vi "fgv_pf-val.vi"(7 "cmd":T4, 11 "pf-val":T3={"DT"=0.0, "SIM_TIME"=0.0, "MAX_RANGE"=0.0, "NP"=0, "NTh"=0, "Q_sim"=[[0.04000000000000001]], "R_sim"=[[1.0, 0.0], [0.0, 0.2741556778080377]]}) -> (3 "pf-val out":T2={"DT"=0.0, "SIM_TIME"=0.0, "MAX_RANGE"=0.0, "NP"=0, "NTh"=0.0, "Q_sim"=[[0.04000000000000001]], "R_sim"=[[1.0, 0.0], [0.0, 0.2741556778080377]]})   [LabVIEW 2019]
uses:
  Ctrl/cmd_common.ctl
  <vilib>/Analysis/Matrix/Datatypes/RealMatrix.ctl
  <vilib>/Analysis/Matrix/NI_Matrix.lvlib
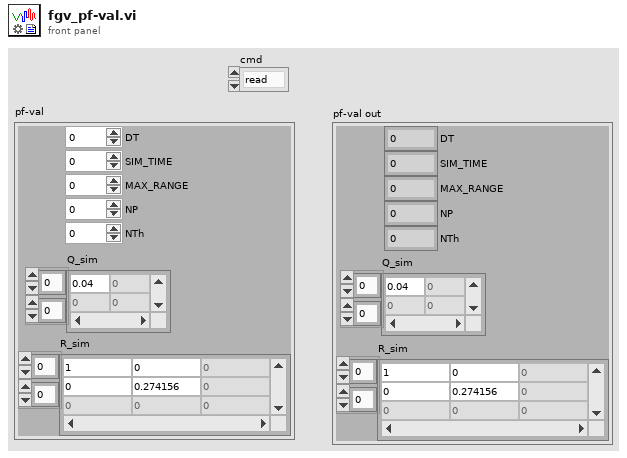
[diagram p1: front panel]
types:
  T1 = typedef "NI_Matrix.lvlib/RealMatrix.ctl" = dbl[][]
  T2 = cluster{"DT":dbl, "SIM_TIME":dbl, "MAX_RANGE":dbl, "NP":u32, "NTh":dbl, "Q_sim":T1, "R_sim":T1}
  T3 = cluster{"DT":dbl, "SIM_TIME":dbl, "MAX_RANGE":dbl, "NP":u32, "NTh":u32, "Q_sim":T1, "R_sim":T1}
  T4 = typedef "cmd_common.ctl" = enum16{"read", "write"}
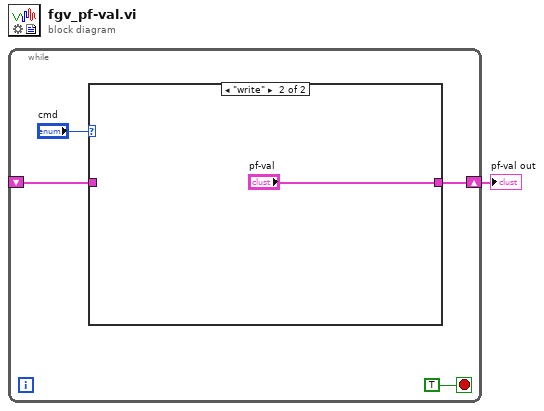
[diagram p0: block diagram]
diagram:
  n1 = while {
    shift-right: [w3] -> w1
    shift-left: _ -> [w2]
    stop <- TRUE stop-if-true
    n2 = case shown="\"write\"" "cmd" {
      tunnel: [w6 "pf-val"] -> w3
      tunnel: w2 -> [w6 _]
      frame "read", Default {
      }
      frame "write" {
      }
    }
  }
  "pf-val out" <- w1
